vi "Variant_to_Timestamp.vi"(8 "Error in":errorcluster, 11 "Value (in)":variant) -> (0 "Error out":errorcluster, 2 "Value (string)":string, 3 "Value (out)":timestamp)   [LabVIEW 2012]
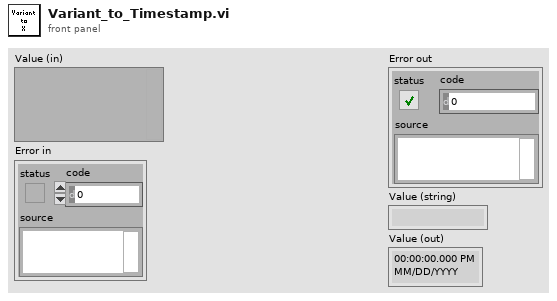
[diagram p1: front panel]
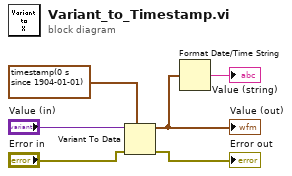
[diagram p0: block diagram]
diagram:
  n1 = Variant To Data(error in="Error in", type=timestamp(0 s since 1904-01-01) ("t0"), Variant="Value (in)") -> (data=w2:timestamp, error out=→"Error out":errorcluster)
  "Value (out)" <- w2
  n2 = Format Date/Time String(seconds (now)=w2) -> (date/time string=→"Value (string)":string)  [unwired: 2 in]
